vi "Image_Crop_Fixed_Area.vi"(6 "Large object threshold":i16, 8 "Particle Measurements in":dbl[][](array[numeric]), 9 "Image  in":T1, 11 "Object size threshold":i32=500) -> (0 "Object accept":bool, 1 "Object":bool, 3 "Crop coordinates array":i32[](array[numeric]))   [LabVIEW 2019]
uses:
  <vilib>/vision/Image Controls.llb/IMAQ Image.ctl
panel:
  out "error out":errorcluster={"status"=TRUE, "code"=-1074396120, "source"="IMAQ Get Image Size\n  "}
  out "Image size/2":i32
  out "Max x":i32
  out "Max y":i32
  in  "Image Border":i32=20
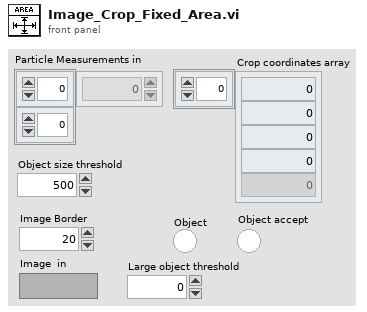
[diagram p1: front panel]
types:
  T1 = typedef "IMAQ Image.ctl" = refnum<image>
  T2 = cluster{"Global Rectangle":i32[], "Contours":cluster{"ID":enum32{"External", "Internal"}, "Type":u32, "Coordinates":i32[]}[]}
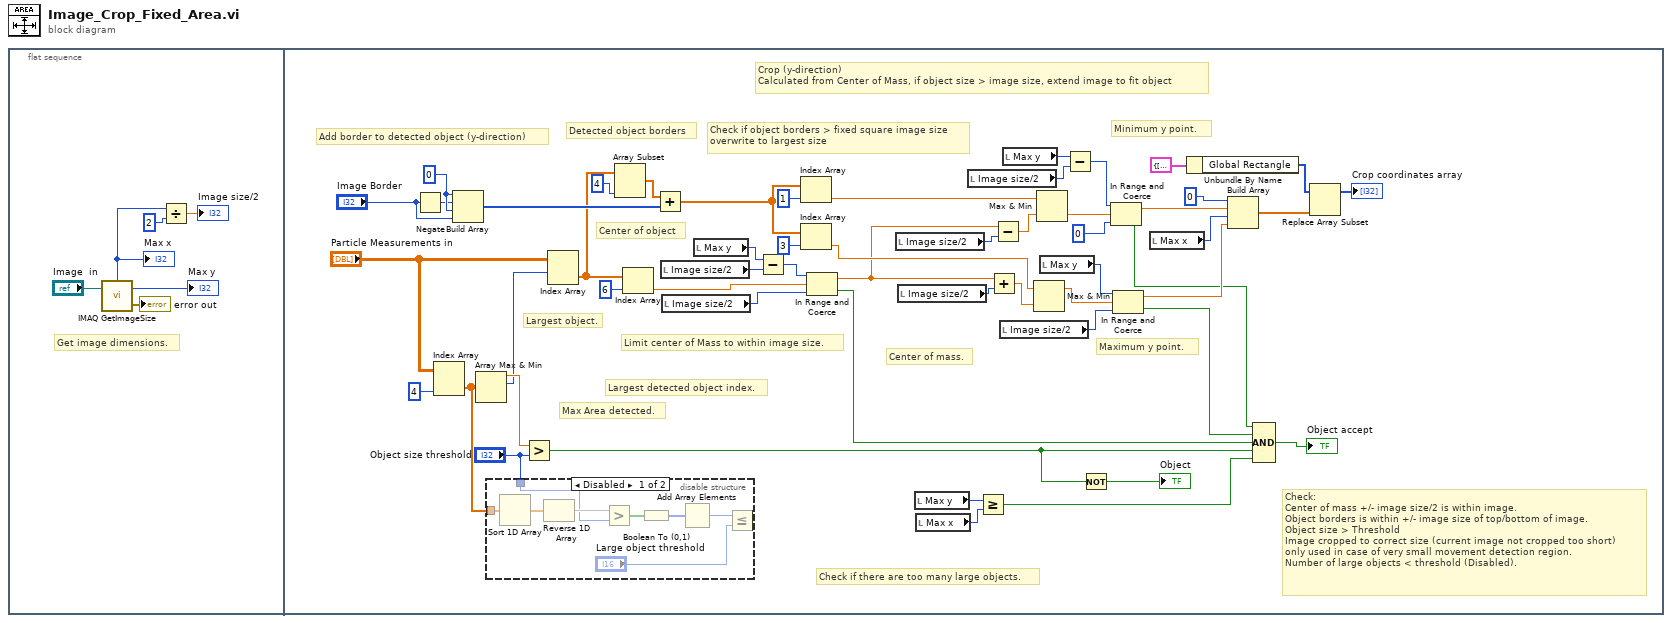
[diagram p0: block diagram]
diagram:
  n1 = flat-sequence {
    frame #0 {
      # "Get image dimensions."
      n2 = call "IMAQ GetImageSize"("Image"="Image  in") -> ("Y Resolution"=→"Max y":i32, "X Resolution"=w4:i32, "error out"=→"error out":errorcluster)  [unwired: 3 in]
      "Max x" <- w4
      n3 = Divide(x=w4, y=2) -> (x/y=→"Image size/2":dbl)
    }
    frame #1 {
      w46 = 0 ("element")
      # "Largest object."
      # "Check if there are too many large objects."
      # "Check:\nCenter of mass +/- image size/2 is within image.\nObject borders is within +/- image size of top/bottom of image.\nObject size > Threshold\nImage cropped to correct size (current image not cropped too short)\nonly used in case of very small movement detection region.\nNumber of large objects < threshold (Disabled)."
      # "Max Area detected."
      # "Maximum y point."
      # "Minimum y point."
      # "Center of mass."
      # "Limit center of Mass to within image size."
      # "Add border to detected object (y-direction)"
      # "Largest detected object index."
      # "Check if object borders > fixed square image size\noverwrite to largest size"
      # "Detected object borders"
      # "Center of object"
      # "Crop (y-direction)\nCalculated from Center of Mass, if object size > image size, extend image to fit object"
      n4 = Negate(x="Image Border") -> (-x=w44:i32)
      n5 = Index Array(array="Particle Measurements in", index (col)=4 ("index (row)")) -> (element=w8:dbl[])  [unwired: 1 in]
      n6 = Build Array(w46, w44, w46, "Image Border") -> (w43:i32[])
      n7 = Array Max & Min(array=w8) -> (max value=w55:dbl, max index (indices)=w53:i32)  [unwired: 2 out]
      n8 = disable-structure shown="Disabled" {
        disable-tunnel: w8 -> [w68 _]
        disable-tunnel: "Object size threshold" -> [w65 _]
        frame Disabled {
          n9 = Sort 1D Array(array=w68) -> (sorted array=w67:dbl[])
          n10 = Reverse 1D Array(array=w67) -> (reversed array=w66:dbl[])
          n11 = Greater?(x=w66, y=w65) -> (0:w64:bool[])
          n12 = Boolean To (0,1)(Boolean=w64) -> (0, 1=w63:i16[])
          n13 = Add Array Elements(numeric array=w63) -> (sum=w62:i16)
          n14 = Less Or Equal?(x=w62, y="Large object threshold") -> ()  [unwired: 1 out]
        }
        frame Enabled {
        }
      }
      n15 = Greater?(x=w55, y="Object size threshold") -> (0:w10:bool)
      n16 = Index Array(array="Particle Measurements in", index (row)=w53) -> (element=w15:dbl[])  [unwired: 1 in]
      n17 = Array Subset(array=w15, length=4) -> (w51:dbl[])  [unwired: 1 in]
      n18 = Index Array(array=w15, index=6) -> (element=w33:dbl)
      n19 = Add(x=w51, y=w43) -> (x+y=w14:dbl[])
      n20 = local read "Image size/2"() -> (w38:i32)
      n21 = local read "Image size/2"() -> (w31:i32)
      n22 = local read "Max y"() -> (w39:i32)
      n23 = Subtract(x=w39, y=w38) -> (x-y=w32:i32)
      n24 = Index Array(array=w14, index=1) -> (element=w49:dbl)
      n25 = Index Array(array=w14, index=3) -> (element=w47:dbl)
      n26 = In Range and Coerce(upper limit=w32, x=w33, lower limit=w31) -> (coerced(x)=w29:dbl, In Range?=w30:bool)
      n27 = local read "Image size/2"() -> (w35:i32)
      n28 = local read "Image size/2"() -> (w34:i32)
      n29 = local read "Max y"() -> (w13:i32)
      n30 = local read "Max x"() -> (w12:i32)
      n31 = local read "Image size/2"() -> (w24:i32)
      n32 = Greater Or Equal?(x=w13, y=w12) -> (x >= y?=w11:bool)
      n33 = Add(x=w29, y=w34) -> (x+y=w37:dbl)
      n34 = Subtract(x=w29, y=w35) -> (x-y=w36:dbl)
      n35 = local read "Image size/2"() -> (w21:i32)
      n36 = local read "Max y"() -> (w25:i32)
      n37 = Max & Min(x=w47, y=w37) -> (max(x,y)=w16:dbl)  [unwired: 1 out]
      n38 = Max & Min(x=w49, y=w36) -> (min(x,y)=w28:dbl)  [unwired: 1 out]
      n39 = local read "Max y"() -> (w22:i32)
      n40 = Subtract(x=w25, y=w24) -> (x-y=w23:i32)
      n41 = Not(x=w10) -> (.not. x?=→"Object":bool)
      n42 = In Range and Coerce(upper limit=w23, x=w28, lower limit=0 ("x")) -> (coerced(x)=w26:dbl, In Range?=w18:bool)
      n43 = In Range and Coerce(upper limit=w22, x=w16, lower limit=w21) -> (coerced(x)=w20:dbl, In Range?=w19:bool)
      n44 = local read "Max x"() -> (w40:i32)
      n45 = Unbundle By Name(T2 {"Global Rectangle"=[106, 29, 356, 265], "Contours"=[{"ID"=enum."External", "Type"=3, "Coordinates"=[106, 29, 356, 265]}]} ("Crop to object")) -> ("Global Rectangle"=w59:i32[])
      n46 = Build Array(0 ("x"), w26, w40, w20) -> (w42:dbl[])
      n47 = Compound Arithmetic op=AND(w18, w19, w30, w10, w11) -> (→"Object accept":bool)
      n48 = Replace Array Subset(array=w59, new element=w42) -> (→"Crop coordinates array":i32[])  [unwired: 1 in]
    }
  }
